vi "Handle Command.vi"(8 "error in (no error)":errorcluster, 9 "Data":variant, 10 "Command":string, 11 "Instrument.Example in":refnum<class "Instrument.Example.lvclass">) -> (0 "error out":errorcluster, 1 "Processed Data":variant, 2 "Command":string, 3 "Instrument.Example out":refnum<class "Instrument.Example.lvclass">)   [LabVIEW 2016, in "Instrument.Example.lvclass"]
uses:
  Instrument.Example.lvclass
  Instrument.Example.lvclass/Instrument.Example.ctl
  <userlib>/LevyLab/Levylab Instruments/SMOs/Instrument/Instrument.lvclass
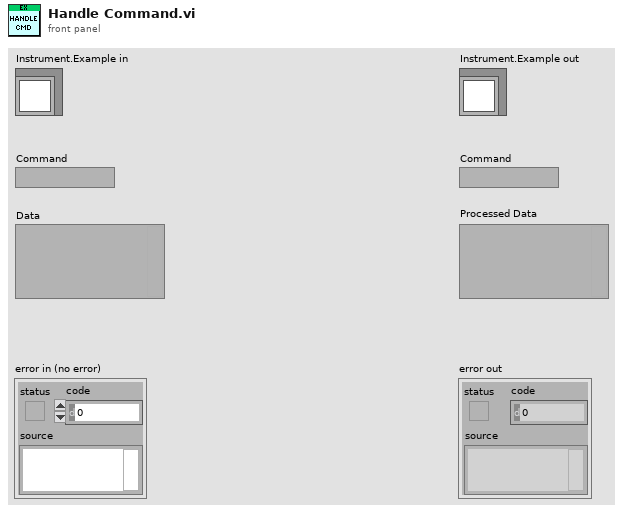
[diagram p1: front panel]
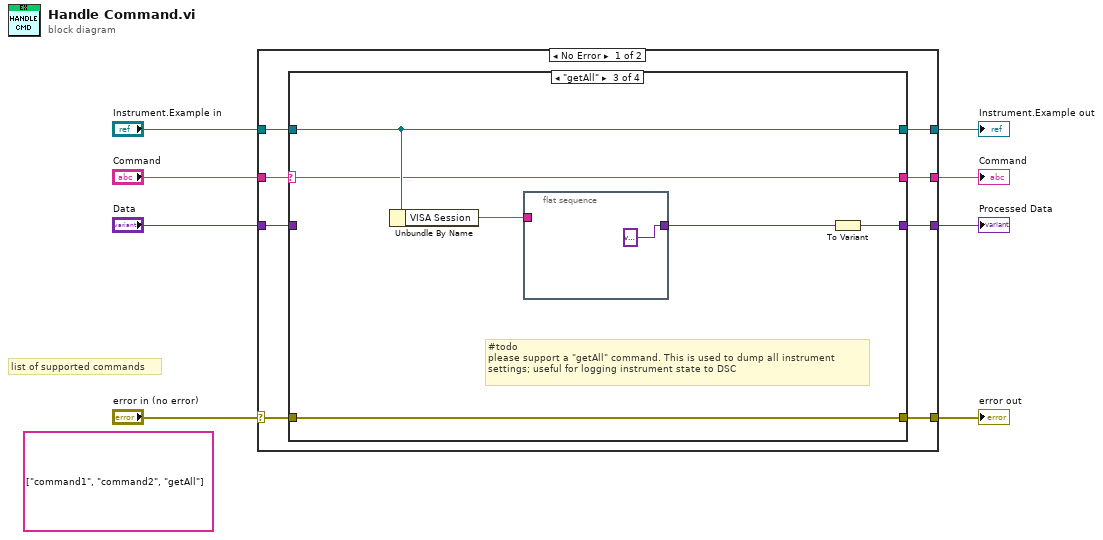
[diagram p0: block diagram]
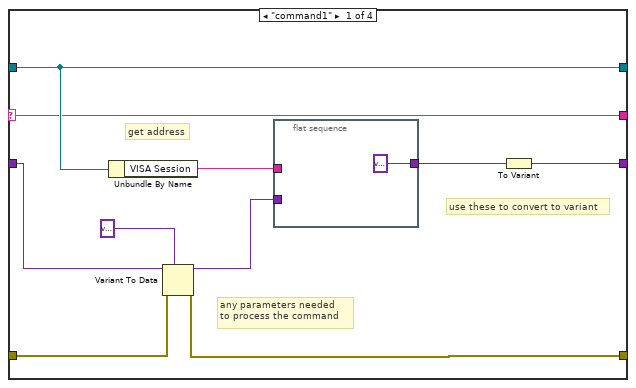
[diagram p2: hidden frame]
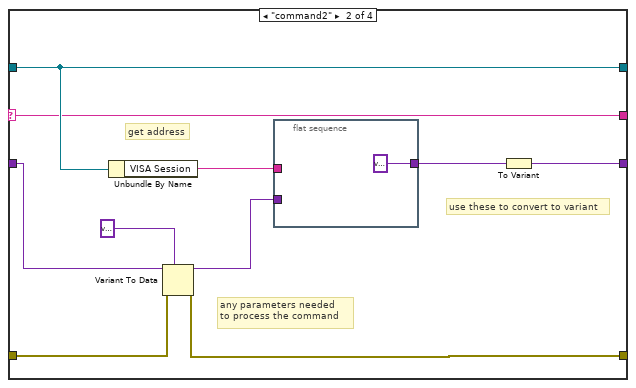
[diagram p3: hidden frame]
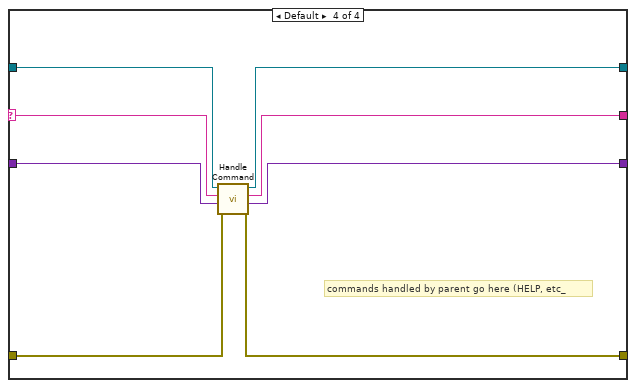
[diagram p4: hidden frame]
diagram:
  (unwired) string[] ["command1", "command2", "getAll"] ("element")
  # "list of supported commands"
  n1 = case shown="No Error" "error in (no error)" {
    selector: "error in (no error)" -> [w11 w54]
    tunnel: [w10 w54] -> w8
    tunnel: [w16 _] -> w7
    tunnel: [w15 _] -> w6
    tunnel: [w14 w55] -> w5
    tunnel: "Data" -> [w13 _]
    tunnel: "Command" -> [w9 _]
    tunnel: "Instrument.Example in" -> [w12 w55]
    frame No Error {
      n2 = case shown="\"getAll\"" w9 {
        selector: w9 -> [w17 w28 w43 w46]
        tunnel: [w21 w32 w42 w53] -> w16
        tunnel: [w17 w28 w43 w52] -> w15
        tunnel: [w25 w36 w44 w51] -> w14
        tunnel: w13 -> [w26 w37 _ w50]
        tunnel: w12 -> [w25 w36 w44 w49]
        tunnel: w11 -> [w24 w35 w41 w48]
        tunnel: [w20 w31 w41 w47] -> w10
        frame "command1" {
          # "use these to convert to variant"
          # "any parameters needed\nto process the command"
          # "get address"
          n3 = Unbundle By Name(w25) -> ("VISA Session"=w19:string)
          n4 = Variant To Data(error in=w24, type=variant ("Data"), Variant=w26) -> (data=w18:variant, error out=w20:errorcluster)
          n5 = flat-sequence {
            tunnel: [variant ("Processed Data")] -> w22
            tunnel: w19 -> [_]
            tunnel: w18 -> [_]
            frame #0 {
            }
          }
          n6 = To Variant(anything=w22) -> (Variant=w21:variant)
        }
        frame "command2" {
          # "use these to convert to variant"
          # "any parameters needed\nto process the command"
          # "get address"
          n7 = Unbundle By Name(w36) -> ("VISA Session"=w30:string)
          n8 = Variant To Data(error in=w35, type=variant ("Data"), Variant=w37) -> (data=w29:variant, error out=w31:errorcluster)
          n9 = flat-sequence {
            tunnel: [variant ("Processed Data")] -> w33
            tunnel: w30 -> [_]
            tunnel: w29 -> [_]
            frame #0 {
            }
          }
          n10 = To Variant(anything=w33) -> (Variant=w32:variant)
        }
        frame "getAll" {
          # "#todo\nplease support a \"getAll\" command. This is used to dump all instrument\nsettings; useful for logging instrument state to DSC"
          n11 = Unbundle By Name(w44) -> ("VISA Session"=w40:string)
          n12 = flat-sequence {
            tunnel: w40 -> [_]
            tunnel: [variant ("Processed Data")] -> w39
            frame #0 {
            }
          }
          n13 = To Variant(anything=w39) -> (Variant=w42:variant)
        }
        frame Default {
          # "commands handled by parent go here (HELP, etc_"
          n14 = call-parent "Handle Command.vi"("error in (no error)"=w48, "Data"=w50, "Command"=w46, "Instrument in"=w49) -> ("error out"=w47:errorcluster, "Processed Data"=w53:variant, "Command"=w52:string, "Instrument out"=w51:refnum<class "Instrument.Example.lvclass">)  [unwired: 4 in]
        }
      }
    }
    frame Error {
    }
  }
  "error out" <- w8
  "Instrument.Example out" <- w5
  "Processed Data" <- w7
  "Command" <- w6
